vi "Replace Array Elements - double.vi"(4 "new elements (none)":dbl[](array[numeric])=[999.0, nan], 5 "indices (none)":i32[](array[numeric])=[3, 5], 7 "1D Array":dbl[](array[numeric])=[0.0, 1.0, 2.0, 3.0, 4.0, 5.0, 6.0, 7.0]) -> (2 "output array":dbl[](array[numeric]))   [LabVIEW 2020]
doc: "Replaces elements in a 1-dim array at the specified indices. This is a list-based version of the built-in \"Replace Array Subset\"."
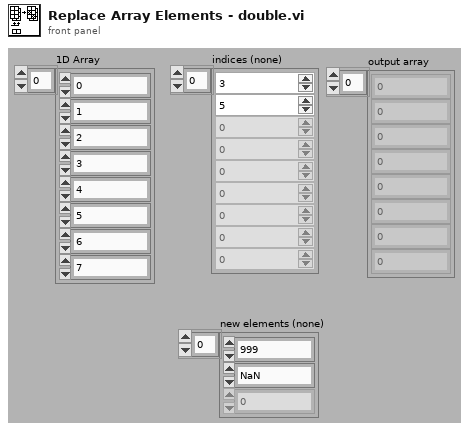
[diagram p1: front panel]
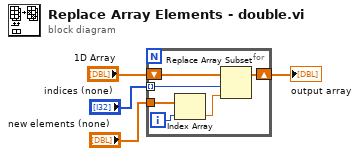
[diagram p0: block diagram]
diagram:
  n1 = for {
    tunnel: "new elements (none)" -> [w8]
    shift-right: [w9] -> w3
    shift-left: "1D Array" -> [w10]
    tunnel: "indices (none)" -> [w6] mode=indexing
    i -> [w5]
    n2 = Index Array(array=w8, index=w5) -> (element=w7:dbl)
    n3 = Replace Array Subset(array=w10, new element=w7, index=w6) -> (w9:dbl[])
  }
  "output array" <- w3
